vi "Set OD Entry Values.vi"(8 "error in":errorcluster, 10 "Values":T1(array[cluster]) {"Multiplexer"."Index" format="%x"}, 11 "Object Dictionary UI in":refnum<class "Object Dictionary UI.lvclass">) -> (0 "error out":errorcluster, 3 "Object Dictionary UI out":refnum<class "Object Dictionary UI.lvclass">)   [LabVIEW 2021, in "Object Dictionary UI.lvlib" / "Object Dictionary UI.lvclass"]
uses:
  Object Dictionary UI.lvclass
  Object Dictionary UI.lvclass/Object Dictionary UI.ctl
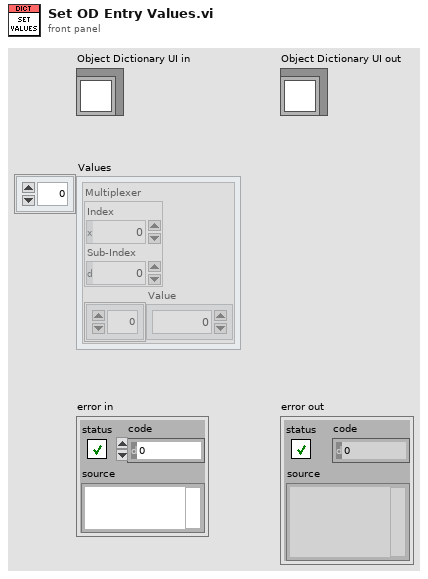
[diagram p1: front panel]
types:
  T1 = cluster{"Multiplexer":cluster{"Index":u16, "Sub-Index":i16}, "Value":u8[]}[]
  T2 = enum16{"UNKNOWN", "BOOLEAN", "INTEGER8", "INTEGER16", "INTEGER32", "UNSIGNED8", "UNSIGNED16", "UNSIGNED32", "REAL32", "VISIBLE_STRING", "OCTET_STRING", "UNICODE_STRING", "TIME_OF_DAY", "TIME_DIFFERENCE", "RESERVED1", "DOMAIN", "INTEGER24", "REAL64", "INTEGER40", "INTEGER48", "INTEGER56", "INTEGER64", "UNSIGNED24", "RESERVED2", "UNSIGNED40", "UNSIGNED48", "UNSIGNED56", "UNSIGNED64", "RESERVED3", "RESERVED4", "RESERVED5", "RESERVED6", "PDO_COMMUNICATION_PARAMETER", "PDO_MAPPING", "SDO_PARAMETER", "IDENTITY", "RESERVED7"}
  T3 = enum16{"ro", "wo", "rw", "rwr", "rww", "const", "UNKNOWN"}
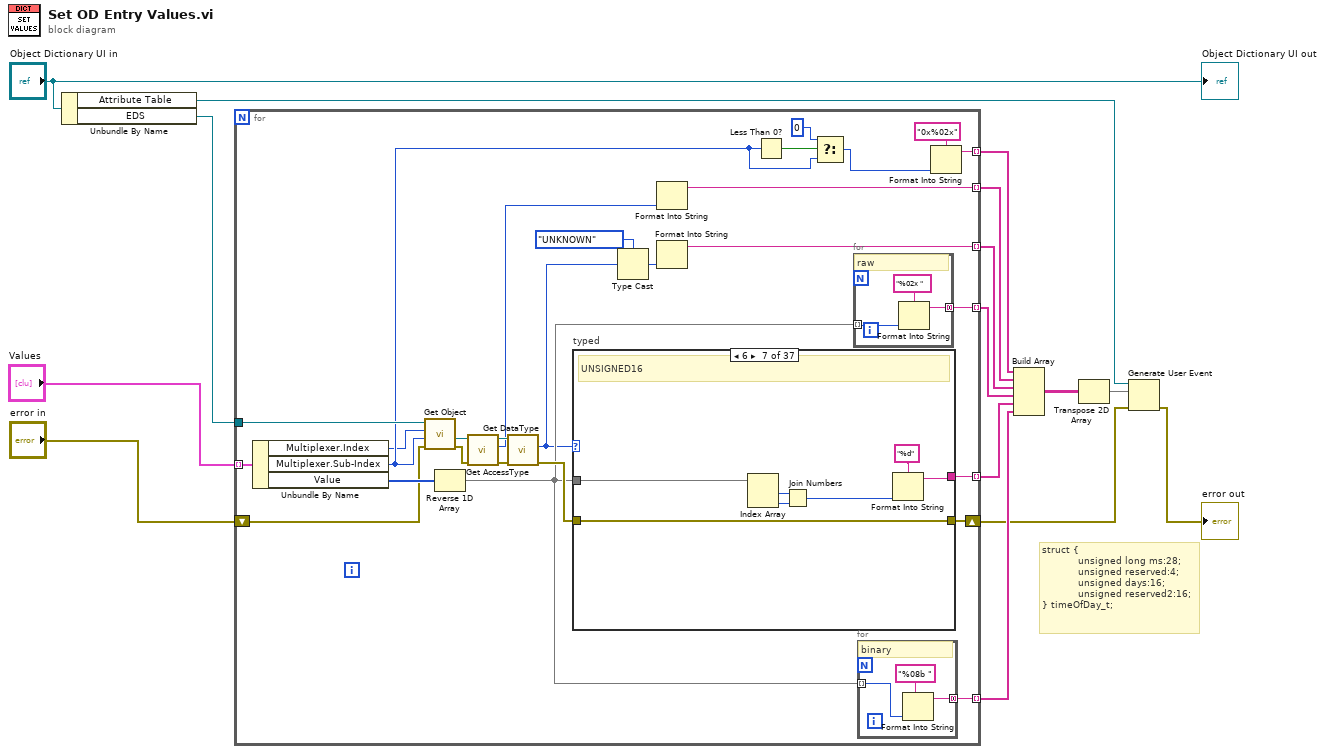
[diagram p0: block diagram]
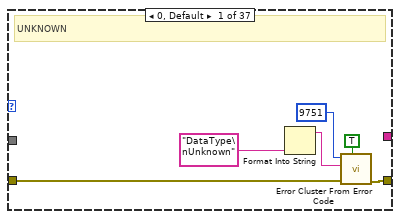
[diagram p2: hidden frame]
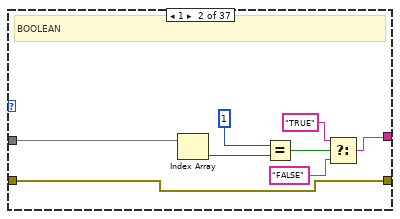
[diagram p3: hidden frame]
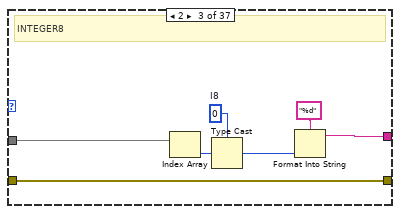
[diagram p4: hidden frame]
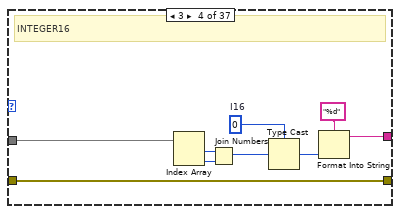
[diagram p5: hidden frame]
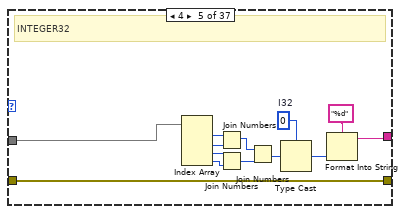
[diagram p6: hidden frame]
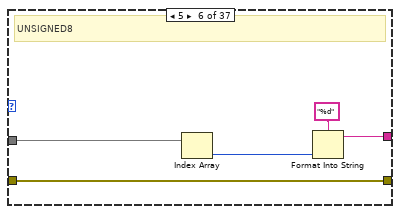
[diagram p7: hidden frame]
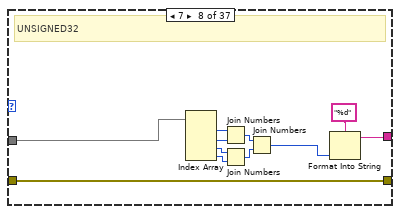
[diagram p8: hidden frame]
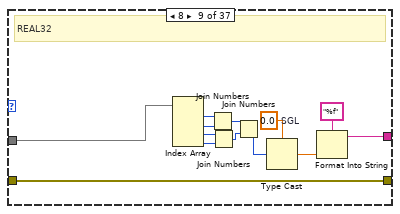
[diagram p9: hidden frame]
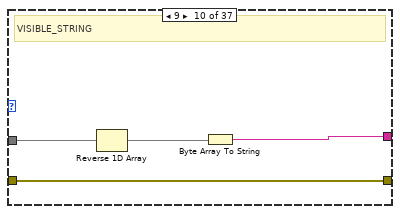
[diagram p10: hidden frame]
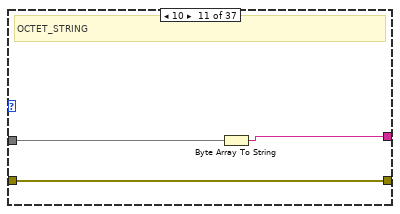
[diagram p11: hidden frame]
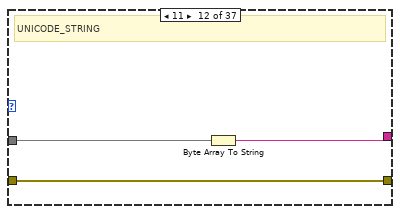
[diagram p12: hidden frame]
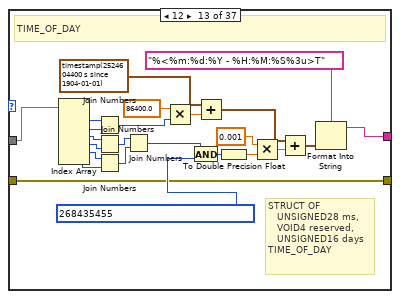
[diagram p13: hidden frame]
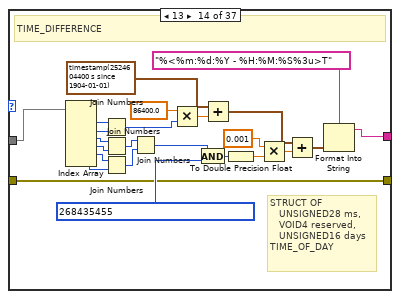
[diagram p14: hidden frame]
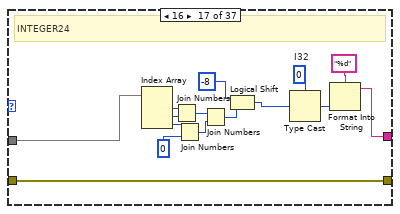
[diagram p17: hidden frame]
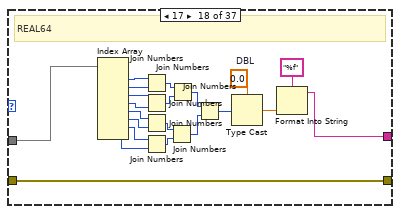
[diagram p18: hidden frame]
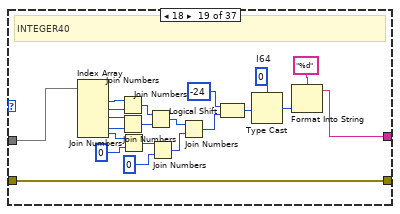
[diagram p19: hidden frame]
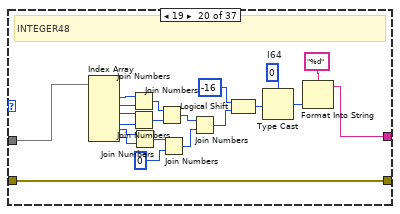
[diagram p20: hidden frame]
diagram:
  # "struct {\n            unsigned long ms:28;\n            unsigned reserved:4;\n            unsigned days:16;\n            unsigned reserved2:16;\n} timeOfDay_t;"
  n1 = Unbundle By Name("Object Dictionary UI in") -> ("Attribute Table"=w6:refnum<user-event>, "EDS"=w13:refnum<class "Electronic Datasheet.lvclass">)
  n2 = for {
    tunnel: "Values" -> [w42] mode=indexing
    tunnel: [w40] -> w3 mode=indexing
    tunnel: w13 -> [w39]
    tunnel: [w38] -> w8 mode=indexing
    shift-right: [w37] -> w5
    shift-left: "error in" -> [w33]
    tunnel: [w36] -> w10 mode=indexing
    tunnel: [w34] -> w9 mode=indexing
    tunnel: [w26] -> w2 mode=indexing
    tunnel: [w20] -> w1 mode=indexing
    n3 = Unbundle By Name(w42) -> ("Multiplexer.Index"=w16:u16, "Multiplexer.Sub-Index"=w28:i16, "Value"=w35:u8[])
    n4 = call "Get Object.vi"("error in"=w33, "Sub-Index"=w28, "Index"=w16, "reference in"=w39) -> ("error out"=w21:errorcluster, "OD Entry"=w25:refnum<class "OD Entry.lvclass">)  [unwired: 4 in, 2 out]
    n5 = Reverse 1D Array(array=w35) -> (reversed array=w27:u8[])
    n6 = call "Get AccessType.vi"("Error In"=w21, "reference in"=w25) -> ("Error Out"=w22:errorcluster, "AccessType"=w23:T3, "reference out"=w24:refnum<class "OD Entry.lvclass">)  [unwired: 7 in]
    n7 = call "Get DataType.vi"("Error In"=w22, "reference in"=w24) -> ("Error Out"=w32:errorcluster, "DataType"=w19:u16)  [unwired: 7 in, 1 out]
    n8 = case "typed" shown="6" w19 {
      tunnel: w27 -> [_ w62 w69 w75 w85 w96 w99 w110 w122 w131 w134 w137 w161 w165 _ _ w199 w218 w224 w248 w271 w295 w314 _ w326 w347 w365 w385 _ _ _ _ _ _ _ _ _]
      tunnel: [_ w56 w65 w76 w86 w93 w98 w111 w116 w130 w133 w136 w142 w166 _ _ w197 w204 w226 w246 w267 w290 w311 _ w324 w345 w363 w383 _ _ _ _ _ _ _ _ _] -> w38
      tunnel: [w50 w55 w63 w70 w79 w92 w97 w104 w115 w129 w132 w135 w138 w162 w186 w187 w188 w203 w225 w249 w266 w289 w310 w323 w342 w346 w382 w386 w402 w403 w404 w405 w406 w407 w408 w409 w410] -> w37
      tunnel: w32 -> [w49 w55 w63 w70 w79 w92 w97 w104 w115 w129 w132 w135 w138 w162 w186 w187 w188 w203 w225 w249 w266 w289 w310 w323 w342 w346 w382 w386 w402 w403 w404 w405 w406 w407 w408 w409 w410]
      frame 0, Default {
        # "UNKNOWN"
        n9 = Format Into String("DataType\nUnknown" ("source")) -> (resulting string=w54:string)  [unwired: 3 in, 1 out]
        n10 = call <vilib>:"Error Cluster From Error Code.vi"("show call chain? (False)"=TRUE, "error in (no error)"=w49, "error message (\"\")"=w54, "error code (0)"=9751) -> ("error out"=w50:errorcluster)  [unwired: 5 in]
      }
      frame 1 {
        # "BOOLEAN"
        n11 = Index Array(array=w62) -> (element=w61:u8)  [unwired: 1 in]
        n12 = Equal?(x=u8 1, y=w61) -> (x = y?=w59:bool)
        n13 = Select(t="TRUE", s=w59, f="FALSE") -> (s? t:f=w56:string)
      }
      frame 2 {
        w64 = i8 0  # I8
        # "INTEGER8"
        n14 = Index Array(array=w69) -> (element=w68:u8)  [unwired: 1 in]
        n15 = Type Cast(type=w64, x=w68) -> (*(type *) &x=w67:i8)
        n16 = Format Into String(format string="%d", w67) -> (resulting string=w65:string)  [unwired: 2 in, 1 out]
      }
      frame 3 {
        w71 = i16 0  # I16
        # "INTEGER16"
        n17 = Index Array(array=w75) -> (element #1=w72:u8, element #2=w73:u8)  [unwired: 2 in]
        n18 = Join Numbers(hi=w72, lo=w73) -> ((hi.lo)=w74:u16)
        n19 = Type Cast(type=w71, x=w74) -> (*(type *) &x=w78:i16)
        n20 = Format Into String(format string="%d", w78) -> (resulting string=w76:string)  [unwired: 2 in, 1 out]
      }
      frame 4 {
        w87 = i16 0  # I32
        # "INTEGER32"
        n21 = Index Array(array=w85) -> (element #1=w88:u8, element #2=w89:u8, element #3=w84:u8, element #4=w83:u8)  [unwired: 4 in]
        n22 = Join Numbers(hi=w88, lo=w89) -> ((hi.lo)=w81:u16)
        n23 = Join Numbers(hi=w84, lo=w83) -> ((hi.lo)=w82:u16)
        n24 = Join Numbers(hi=w81, lo=w82) -> ((hi.lo)=w80:u32)
        n25 = Type Cast(type=w87, x=w80) -> (*(type *) &x=w91:i16)
        n26 = Format Into String(format string="%d", w91) -> (resulting string=w86:string)  [unwired: 2 in, 1 out]
      }
      frame 5 {
        # "UNSIGNED8"
        n27 = Index Array(array=w96) -> (element=w95:u8)  [unwired: 1 in]
        n28 = Format Into String(format string="%d", w95) -> (resulting string=w93:string)  [unwired: 2 in, 1 out]
      }
      frame 6 {
        # "UNSIGNED16"
        n29 = Index Array(array=w99) -> (element #1=w100:u8, element #2=w101:u8)  [unwired: 2 in]
        n30 = Join Numbers(hi=w100, lo=w101) -> ((hi.lo)=w102:u16)
        n31 = Format Into String(format string="%d", w102) -> (resulting string=w98:string)  [unwired: 2 in, 1 out]
      }
      frame 7 {
        # "UNSIGNED32"
        n32 = Index Array(array=w110) -> (element #1=w112:u8, element #2=w113:u8, element #3=w106:u8, element #4=w107:u8)  [unwired: 4 in]
        n33 = Join Numbers(hi=w112, lo=w113) -> ((hi.lo)=w109:u16)
        n34 = Join Numbers(hi=w106, lo=w107) -> ((hi.lo)=w108:u16)
        n35 = Join Numbers(hi=w109, lo=w108) -> ((hi.lo)=w105:u32)
        n36 = Format Into String(format string="%d", w105) -> (resulting string=w111:string)  [unwired: 2 in, 1 out]
      }
      frame 8 {
        w123 = sgl 0.0  # SGL
        # "REAL32"
        n37 = Index Array(array=w122) -> (element #1=w124:u8, element #2=w125:u8, element #3=w121:u8, element #4=w120:u8)  [unwired: 4 in]
        n38 = Join Numbers(hi=w124, lo=w125) -> ((hi.lo)=w118:u16)
        n39 = Join Numbers(hi=w121, lo=w120) -> ((hi.lo)=w119:u16)
        n40 = Join Numbers(hi=w118, lo=w119) -> ((hi.lo)=w117:u32)
        n41 = Type Cast(type=w123, x=w117) -> (*(type *) &x=w127:sgl)
        n42 = Format Into String(format string="%f", w127) -> (resulting string=w116:string)  [unwired: 2 in, 1 out]
      }
      frame 9 {
        # "VISIBLE_STRING"
        n43 = Reverse 1D Array(array=w131) -> (reversed array=w128:u8[])
        n44 = Byte Array To String(unsigned byte array=w128) -> (string=w130:string)
      }
      frame 10 {
        # "OCTET_STRING"
        n45 = Byte Array To String(unsigned byte array=w134) -> (string=w133:string)
      }
      frame 11 {
        # "UNICODE_STRING"
        n46 = Byte Array To String(unsigned byte array=w137) -> (string=w136:string)
      }
      frame 12 {
        # "STRUCT OF\n   UNSIGNED28 ms,\n   VOID4 reserved,\n   UNSIGNED16 days\nTIME_OF_DAY"
        # "TIME_OF_DAY"
        n47 = Index Array(array=w161) -> (element #1=w160:u8, element #2=w159:u8, element #3=w154:u8, element #4=w153:u8, element #5=w152:u8, element #6=w151:u8)  [unwired: 6 in]
        n48 = Join Numbers(hi=w160, lo=w159) -> ((hi.lo)=w155:u16)
        n49 = Join Numbers(hi=w154, lo=w153) -> ((hi.lo)=w150:u16)
        n50 = Join Numbers(hi=w152, lo=w151) -> ((hi.lo)=w149:u16)
        n51 = Join Numbers(hi=w150, lo=w149) -> ((hi.lo)=w148:u32)
        n52 = Multiply(x=86400.0, y=w155) -> (x*y=w157:dbl)
        n53 = And(x=w148, y=u32 268435455) -> (x .and. y?=w147:u32)
        n54 = Add(x=timestamp(2524604400 s since 1904-01-01), y=w157) -> (x+y=w143:timestamp)
        n55 = To Double Precision Float(number=w147) -> (double precision float=w146:dbl)
        n56 = Multiply(x=0.001, y=w146) -> (x*y=w144:dbl)
        n57 = Add(x=w143, y=w144) -> (x+y=w141:timestamp)
        n58 = Format Into String(format string="%<%m:%d:%Y - %H:%M:%S%3u>T", w141) -> (resulting string=w142:string)  [unwired: 2 in, 1 out]
      }
      frame 13 {
        # "STRUCT OF\n   UNSIGNED28 ms,\n   VOID4 reserved,\n   UNSIGNED16 days\nTIME_OF_DAY"
        # "TIME_DIFFERENCE"
        n59 = Index Array(array=w165) -> (element #1=w185:u8, element #2=w184:u8, element #3=w179:u8, element #4=w178:u8, element #5=w177:u8, element #6=w176:u8)  [unwired: 6 in]
        n60 = Join Numbers(hi=w185, lo=w184) -> ((hi.lo)=w180:u16)
        n61 = Join Numbers(hi=w179, lo=w178) -> ((hi.lo)=w175:u16)
        n62 = Join Numbers(hi=w177, lo=w176) -> ((hi.lo)=w174:u16)
        n63 = Join Numbers(hi=w175, lo=w174) -> ((hi.lo)=w173:u32)
        n64 = Multiply(x=86400.0, y=w180) -> (x*y=w182:dbl)
        n65 = And(x=w173, y=u32 268435455) -> (x .and. y?=w172:u32)
        n66 = Add(x=timestamp(2524604400 s since 1904-01-01), y=w182) -> (x+y=w168:timestamp)
        n67 = To Double Precision Float(number=w172) -> (double precision float=w171:dbl)
        n68 = Multiply(x=0.001, y=w171) -> (x*y=w169:dbl)
        n69 = Add(x=w168, y=w169) -> (x+y=w167:timestamp)
        n70 = Format Into String(format string="%<%m:%d:%Y - %H:%M:%S%3u>T", w167) -> (resulting string=w166:string)  [unwired: 2 in, 1 out]
      }
      frame 14 {
        # "RESERVED1"
      }
      frame 15 {
        # "DOMAIN"
      }
      frame 16 {
        w200 = 0  # I32
        # "INTEGER24"
        n71 = Index Array(array=w199) -> (element #1=w195:u8, element #2=w196:u8, element #3=w194:u8)  [unwired: 3 in]
        n72 = Join Numbers(hi=w195, lo=w196) -> ((hi.lo)=w192:u16)
        n73 = Join Numbers(hi=w194, lo=u8 0) -> ((hi.lo)=w193:u16)
        n74 = Join Numbers(hi=w192, lo=w193) -> ((hi.lo)=w191:u32)
        n75 = Logical Shift(y=i16 -8, x=w191) -> (x << y=w190:u32)
        n76 = Type Cast(type=w200, x=w190) -> (*(type *) &x=w202:i32)
        n77 = Format Into String(format string="%d", w202) -> (resulting string=w197:string)  [unwired: 2 in, 1 out]
      }
      frame 17 {
        w221 = 0.0  # DBL
        # "REAL64"
        n78 = Index Array(array=w218) -> (element #1=w219:u8, element #2=w220:u8, element #3=w217:u8, element #4=w216:u8, element #5=w215:u8, element #6=w214:u8, element #7=w213:u8, element #8=w212:u8)  [unwired: 8 in]
        n79 = Join Numbers(hi=w219, lo=w220) -> ((hi.lo)=w209:u16)
        n80 = Join Numbers(hi=w217, lo=w216) -> ((hi.lo)=w208:u16)
        n81 = Join Numbers(hi=w215, lo=w214) -> ((hi.lo)=w210:u16)
        n82 = Join Numbers(hi=w213, lo=w212) -> ((hi.lo)=w211:u16)
        n83 = Join Numbers(hi=w210, lo=w211) -> ((hi.lo)=w206:u32)
        n84 = Join Numbers(hi=w209, lo=w208) -> ((hi.lo)=w207:u32)
        n85 = Join Numbers(hi=w207, lo=w206) -> ((hi.lo)=w205:u64)
        n86 = Type Cast(type=w221, x=w205) -> (*(type *) &x=w223:dbl)
        n87 = Format Into String(format string="%f", w223) -> (resulting string=w204:string)  [unwired: 2 in, 1 out]
      }
      frame 18 {
        w242 = i64 0  # I64
        # "INTEGER40"
        n88 = Index Array(array=w224) -> (element #1=w239:u8, element #2=w240:u8, element #3=w238:u8, element #4=w237:u8, element #5=w236:u8)  [unwired: 5 in]
        n89 = Join Numbers(hi=w239, lo=w240) -> ((hi.lo)=w233:u16)
        n90 = Join Numbers(hi=w238, lo=w237) -> ((hi.lo)=w234:u16)
        n91 = Join Numbers(hi=w236, lo=u8 0) -> ((hi.lo)=w232:u16)
        n92 = Join Numbers(hi=w233, lo=w234) -> ((hi.lo)=w229:u32)
        n93 = Join Numbers(hi=w232, lo=u16 0) -> ((hi.lo)=w228:u32)
        n94 = Join Numbers(hi=w229, lo=w228) -> ((hi.lo)=w227:u64)
        n95 = Logical Shift(y=i16 -24, x=w227) -> (x << y=w230:u64)
        n96 = Type Cast(type=w242, x=w230) -> (*(type *) &x=w244:i64)
        n97 = Format Into String(format string="%d", w244) -> (resulting string=w226:string)  [unwired: 2 in, 1 out]
      }
      frame 19 {
        w263 = i64 0  # I64
        # "INTEGER48"
        n98 = Index Array(array=w248) -> (element #1=w260:u8, element #2=w261:u8, element #3=w259:u8, element #4=w258:u8, element #5=w257:u8, element #6=w247:u8)  [unwired: 6 in]
        n99 = Join Numbers(hi=w260, lo=w261) -> ((hi.lo)=w255:u16)
        n100 = Join Numbers(hi=w259, lo=w258) -> ((hi.lo)=w256:u16)
        n101 = Join Numbers(hi=w257, lo=w247) -> ((hi.lo)=w254:u16)
        n102 = Join Numbers(hi=w255, lo=w256) -> ((hi.lo)=w252:u32)
        n103 = Join Numbers(hi=w254, lo=u16 0) -> ((hi.lo)=w251:u32)
        n104 = Join Numbers(hi=w252, lo=w251) -> ((hi.lo)=w250:u64)
        n105 = Logical Shift(y=i16 -16, x=w250) -> (x << y=w253:u64)
        n106 = Type Cast(type=w263, x=w253) -> (*(type *) &x=w265:i64)
        n107 = Format Into String(format string="%d", w265) -> (resulting string=w246:string)  [unwired: 2 in, 1 out]
      }
      frame 20 {
        w286 = i64 0  # I64
        # "INTEGER56"
        n108 = Index Array(array=w271) -> (element #1=w283:u8, element #2=w284:u8, element #3=w282:u8, element #4=w281:u8, element #5=w280:u8, element #6=w272:u8, element #7=w269:u8)  [unwired: 7 in]
        n109 = Join Numbers(hi=w283, lo=w284) -> ((hi.lo)=w278:u16)
        n110 = Join Numbers(hi=w282, lo=w281) -> ((hi.lo)=w279:u16)
        n111 = Join Numbers(hi=w280, lo=w272) -> ((hi.lo)=w277:u16)
        n112 = Join Numbers(hi=w269, lo=u8 0) -> ((hi.lo)=w268:u16)
        n113 = Join Numbers(hi=w278, lo=w279) -> ((hi.lo)=w275:u32)
        n114 = Join Numbers(hi=w277, lo=w268) -> ((hi.lo)=w274:u32)
        n115 = Join Numbers(hi=w275, lo=w274) -> ((hi.lo)=w273:u64)
        n116 = Logical Shift(y=i16 -8, x=w273) -> (x << y=w276:u64)
        n117 = Type Cast(type=w286, x=w276) -> (*(type *) &x=w288:i64)
        n118 = Format Into String(format string="%d", w288) -> (resulting string=w267:string)  [unwired: 2 in, 1 out]
      }
      frame 21 {
        w307 = i64 0  # I64
        # "INTEGER64"
        n119 = Index Array(array=w295) -> (element #1=w305:u8, element #2=w306:u8, element #3=w304:u8, element #4=w303:u8, element #5=w302:u8, element #6=w296:u8, element #7=w294:u8, element #8=w293:u8)  [unwired: 8 in]
        n120 = Join Numbers(hi=w305, lo=w306) -> ((hi.lo)=w300:u16)
        n121 = Join Numbers(hi=w304, lo=w303) -> ((hi.lo)=w301:u16)
        n122 = Join Numbers(hi=w302, lo=w296) -> ((hi.lo)=w299:u16)
        n123 = Join Numbers(hi=w294, lo=w293) -> ((hi.lo)=w292:u16)
        n124 = Join Numbers(hi=w300, lo=w301) -> ((hi.lo)=w298:u32)
        n125 = Join Numbers(hi=w299, lo=w292) -> ((hi.lo)=w297:u32)
        n126 = Join Numbers(hi=w298, lo=w297) -> ((hi.lo)=w291:u64)
        n127 = Type Cast(type=w307, x=w291) -> (*(type *) &x=w309:i64)
        n128 = Format Into String(format string="%d", w309) -> (resulting string=w290:string)  [unwired: 2 in, 1 out]
      }
      frame 22 {
        # "UNSIGNED24"
        n129 = Index Array(array=w314) -> (element #1=w320:u8, element #2=w321:u8, element #3=w319:u8)  [unwired: 3 in]
        n130 = Join Numbers(hi=w320, lo=w321) -> ((hi.lo)=w317:u16)
        n131 = Join Numbers(hi=w319, lo=u8 0) -> ((hi.lo)=w318:u16)
        n132 = Join Numbers(hi=w317, lo=w318) -> ((hi.lo)=w316:u32)
        n133 = Logical Shift(y=i16 -8, x=w316) -> (x << y=w312:u32)
        n134 = Format Into String(format string="%d", w312) -> (resulting string=w311:string)  [unwired: 2 in, 1 out]
      }
      frame 23 {
        # "RESERVED2"
      }
      frame 24 {
        # "UNSIGNED40"
        n135 = Index Array(array=w326) -> (element #1=w338:u8, element #2=w339:u8, element #3=w337:u8, element #4=w336:u8, element #5=w335:u8)  [unwired: 5 in]
        n136 = Join Numbers(hi=w338, lo=w339) -> ((hi.lo)=w332:u16)
        n137 = Join Numbers(hi=w337, lo=w336) -> ((hi.lo)=w333:u16)
        n138 = Join Numbers(hi=w335, lo=u8 0) -> ((hi.lo)=w331:u16)
        n139 = Join Numbers(hi=w332, lo=w333) -> ((hi.lo)=w329:u32)
        n140 = Join Numbers(hi=w331, lo=u16 0) -> ((hi.lo)=w328:u32)
        n141 = Join Numbers(hi=w329, lo=w328) -> ((hi.lo)=w327:u64)
        n142 = Logical Shift(y=i16 -24, x=w327) -> (x << y=w325:u64)
        n143 = Format Into String(format string="%d", w325) -> (resulting string=w324:string)  [unwired: 2 in, 1 out]
      }
      frame 25 {
        # "UNSIGNED48"
        n144 = Index Array(array=w347) -> (element #1=w358:u8, element #2=w359:u8, element #3=w357:u8, element #4=w356:u8, element #5=w355:u8, element #6=w348:u8)  [unwired: 6 in]
        n145 = Join Numbers(hi=w358, lo=w359) -> ((hi.lo)=w353:u16)
        n146 = Join Numbers(hi=w357, lo=w356) -> ((hi.lo)=w354:u16)
        n147 = Join Numbers(hi=w355, lo=w348) -> ((hi.lo)=w352:u16)
        n148 = Join Numbers(hi=w353, lo=w354) -> ((hi.lo)=w351:u32)
        n149 = Join Numbers(hi=w352, lo=u16 0) -> ((hi.lo)=w350:u32)
        n150 = Join Numbers(hi=w351, lo=w350) -> ((hi.lo)=w349:u64)
        n151 = Logical Shift(y=i16 -16, x=w349) -> (x << y=w344:u64)
        n152 = Format Into String(format string="%d", w344) -> (resulting string=w345:string)  [unwired: 2 in, 1 out]
      }
      frame 26 {
        # "UNSIGNED56"
        n153 = Index Array(array=w365) -> (element #1=w378:u8, element #2=w379:u8, element #3=w377:u8, element #4=w376:u8, element #5=w375:u8, element #6=w368:u8, element #7=w367:u8)  [unwired: 7 in]
        n154 = Join Numbers(hi=w378, lo=w379) -> ((hi.lo)=w373:u16)
        n155 = Join Numbers(hi=w377, lo=w376) -> ((hi.lo)=w374:u16)
        n156 = Join Numbers(hi=w375, lo=w368) -> ((hi.lo)=w372:u16)
        n157 = Join Numbers(hi=w367, lo=u8 0) -> ((hi.lo)=w366:u16)
        n158 = Join Numbers(hi=w373, lo=w374) -> ((hi.lo)=w371:u32)
        n159 = Join Numbers(hi=w372, lo=w366) -> ((hi.lo)=w370:u32)
        n160 = Join Numbers(hi=w371, lo=w370) -> ((hi.lo)=w369:u64)
        n161 = Logical Shift(y=i16 -8, x=w369) -> (x << y=w364:u64)
        n162 = Format Into String(format string="%d", w364) -> (resulting string=w363:string)  [unwired: 2 in, 1 out]
      }
      frame 27 {
        # "UNSIGNED64"
        n163 = Index Array(array=w385) -> (element #1=w399:u8, element #2=w400:u8, element #3=w398:u8, element #4=w397:u8, element #5=w396:u8, element #6=w390:u8, element #7=w389:u8, element #8=w384:u8)  [unwired: 8 in]
        n164 = Join Numbers(hi=w399, lo=w400) -> ((hi.lo)=w394:u16)
        n165 = Join Numbers(hi=w398, lo=w397) -> ((hi.lo)=w395:u16)
        n166 = Join Numbers(hi=w396, lo=w390) -> ((hi.lo)=w393:u16)
        n167 = Join Numbers(hi=w389, lo=w384) -> ((hi.lo)=w388:u16)
        n168 = Join Numbers(hi=w394, lo=w395) -> ((hi.lo)=w392:u32)
        n169 = Join Numbers(hi=w393, lo=w388) -> ((hi.lo)=w391:u32)
        n170 = Join Numbers(hi=w392, lo=w391) -> ((hi.lo)=w387:u64)
        n171 = Format Into String(format string="%d", w387) -> (resulting string=w383:string)  [unwired: 2 in, 1 out]
      }
      frame 28 {
        # "RESERVED3"
      }
      frame 29 {
        # "RESERVED4"
      }
      frame 30 {
        # "RESERVED5"
      }
      frame 31 {
        # "RESERVED6"
      }
      frame 32 {
        # "PDO_COMMUNICATION_PARAMETER"
      }
      frame 33 {
        # "PDO_MAPPING"
      }
      frame 34 {
        # "SDO_PARAMETER"
      }
      frame 35 {
        # "IDENTITY"
      }
      frame 36 {
        # "RESERVED7"
      }
    }
    n172 = Type Cast(type=T2."UNKNOWN" ("DataType"), x=w19) -> (*(type *) &x=w18:T2)
    n173 = Format Into String(w23) -> (resulting string=w26:string)  [unwired: 3 in, 1 out]
    n174 = Format Into String(w18) -> (resulting string=w20:string)  [unwired: 3 in, 1 out]
    n175 = Less Than 0?(x=w28) -> (x < 0?=w30:bool)
    n176 = Select(t=i16 0, s=w30, f=w28) -> (s? t:f=w31:i16)
    n177 = for {
      tunnel: w27 -> [w47] mode=indexing
      tunnel: [w46] -> w36 mode=concatenating
      # "raw"
      n178 = Format Into String(format string="%02x ", w47) -> (resulting string=w46:string)  [unwired: 2 in, 1 out]
    }
    n179 = for {
      tunnel: w27 -> [w44] mode=indexing
      tunnel: [w43] -> w34 mode=concatenating
      # "binary"
      n180 = Format Into String(format string="%08b ", w44) -> (resulting string=w43:string)  [unwired: 2 in, 1 out]
    }
    n181 = Format Into String(format string="0x%02x", w31) -> (resulting string=w40:string)  [unwired: 2 in, 1 out]
  }
  n182 = Build Array(w3, w2, w1, w10, w8, w9) -> (w12:string[][])
  n183 = Transpose 2D Array(2D array=w12) -> (transposed array=w7:string[][])
  n184 = Generate User Event(user event=w6, event data cluster=w7, error in=w5) -> (error out=→"error out":errorcluster)  [unwired: 1 in, 1 out]
  "Object Dictionary UI out" <- "Object Dictionary UI in"
